vi "Build Camera IP.vi"(8 "Camera Number":i32=9, 11 "Robot IP":string) -> (3 "Camera IP":string)   [LabVIEW 2011]
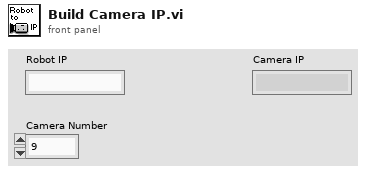
[diagram p1: front panel]
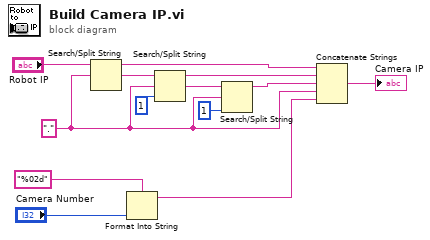
[diagram p0: block diagram]
diagram:
  w4 = "."
  n1 = Search/Split String(string="Robot IP", search string/char (-)=w4) -> (substring before match=w10:string, match + rest of string=w12:string)  [unwired: 1 in, 1 out]
  n2 = Format Into String(format string="%02d", "Camera Number") -> (resulting string=w2:string)  [unwired: 2 in, 1 out]
  n3 = Search/Split String(string=w12, search string/char (-)=w4, offset (0)=1) -> (substring before match=w9:string, match + rest of string=w11:string)  [unwired: 1 out]
  n4 = Search/Split String(string=w11, search string/char (-)=w4, offset (0)=1) -> (substring before match=w8:string)  [unwired: 2 out]
  n5 = Concatenate Strings(w10, w9, w8, w4, w2) -> (→"Camera IP":string)
